vi "C4Buf_writeFeature.vi"(0 "c4buf in":refnum<k24>, 5 "name in":string, 7 "value in":string, 11 "error in":errorcluster) -> (4 "c4buf out":refnum<k24>, 15 "error out":errorcluster)   [LabVIEW 2015, in "libC4HdlLV.lvlib"]
uses:
  libC4HdlLV.lvlib
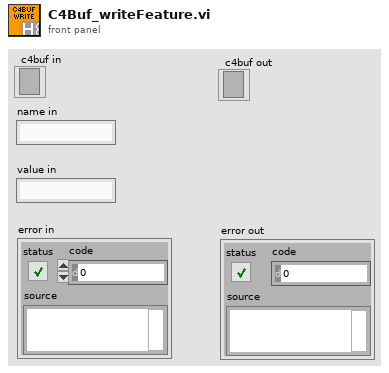
[diagram p1: front panel]
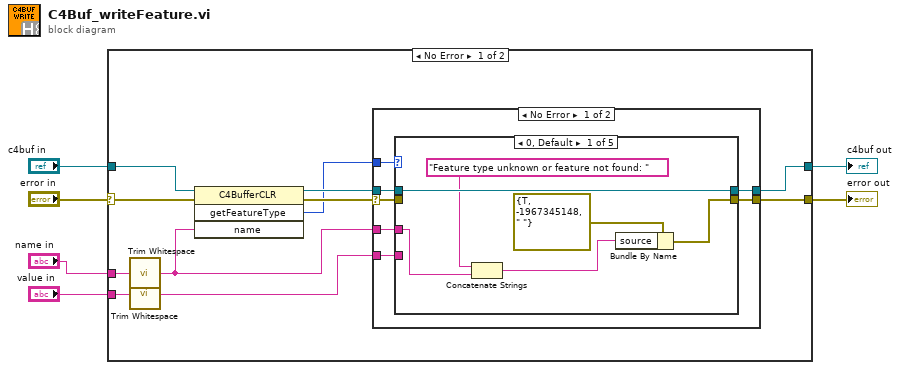
[diagram p0: block diagram]
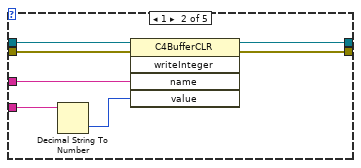
[diagram p2: hidden frame]
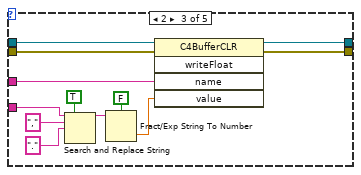
[diagram p3: hidden frame]
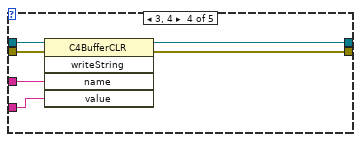
[diagram p4: hidden frame]
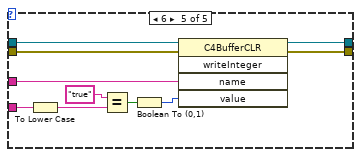
[diagram p5: hidden frame]
diagram:
  n1 = case shown="No Error" "error in" {
    selector: "error in" -> [w11 w69]
    tunnel: [w16 w68] -> w1
    tunnel: [w15 w69] -> w2
    tunnel: "name in" -> [w14 _]
    tunnel: "c4buf in" -> [w12 w68]
    tunnel: "value in" -> [w10 _]
    frame No Error {
      n2 = call <vilib>:"Trim Whitespace.vi"("string"=w14) -> ("trimmed string"=w9:string)  [unwired: 1 in]
      n3 = call <vilib>:"Trim Whitespace.vi"("string"=w10) -> ("trimmed string"=w13:string)  [unwired: 1 in]
      n4 = invoke class="C4BufferCLR" method="getFeatureType"(reference=w12, error in=w11, "name"=w9) -> (reference out=w17:refnum<k24>, error out=w8:errorcluster, "getFeatureType"=w7:i64)  [unwired: 1 in, 1 out]
      n5 = case shown="No Error" w8 {
        selector: w8 -> [w19 w67]
        tunnel: w17 -> [w24 w66]
        tunnel: [w23 w66] -> w16
        tunnel: [w22 w67] -> w15
        tunnel: w13 -> [w21 _]
        tunnel: w9 -> [w20 _]
        tunnel: w7 -> [w18 _]
        frame No Error {
          n6 = case shown="0, Default" w18 {
            tunnel: w24 -> [w30 w37 w49 w55 w65]
            tunnel: w19 -> [_ w36 w48 w54 w64]
            tunnel: w20 -> [w27 w33 w46 w53 w63]
            tunnel: w21 -> [_ w35 w42 w50 w60]
            tunnel: [w30 w32 w45 w52 w62] -> w23
            tunnel: [w25 w31 w44 w51 w61] -> w22
            frame 0, Default {
              n7 = Concatenate Strings("Feature type unknown or feature not found: " ("source"), w27) -> (w29:string)
              n8 = Bundle By Name(cluster=errorcluster {"status"=TRUE, "code"=-1967345148, "source"=" "} ("error out"), "source"=w29) -> (w25:errorcluster)
            }
            frame 1 {
              n9 = Decimal String To Number(string=w35) -> (number=w34:i32)  [unwired: 2 in, 1 out]
              n10 = invoke class="C4BufferCLR" method="writeInteger"(reference=w37, error in=w36, "name"=w33, "value"=w34) -> (reference out=w32:refnum<k24>, error out=w31:errorcluster)  [unwired: 1 in, 3 out]
            }
            frame 2 {
              n11 = Search and Replace String(replace all?=TRUE ("replace all? (F)"), input string=w42, search string=",", replace string="." ("replace string (\"\")")) -> (result string=w41:string)  [unwired: 4 in, 3 out]
              n12 = Fract/Exp String To Number(use system decimal point (T)=FALSE, string=w41) -> (number=w47:dbl)  [unwired: 2 in, 1 out]
              n13 = invoke class="C4BufferCLR" method="writeFloat"(reference=w49, error in=w48, "name"=w46, "value"=w47) -> (reference out=w45:refnum<k24>, error out=w44:errorcluster)  [unwired: 1 in, 3 out]
            }
            frame 3, 4 {
              n14 = invoke class="C4BufferCLR" method="writeString"(reference=w55, error in=w54, "name"=w53, "value"=w50) -> (reference out=w52:refnum<k24>, error out=w51:errorcluster)  [unwired: 1 in, 3 out]
            }
            frame 6 {
              n15 = To Lower Case(string=w60) -> (all lower case string=w59:string)
              n16 = Equal?(x="true", y=w59) -> (x = y?=w56:bool)
              n17 = Boolean To (0,1)(Boolean=w56) -> (0, 1=w57:i16)
              n18 = invoke class="C4BufferCLR" method="writeInteger"(reference=w65, error in=w64, "name"=w63, "value"=w57) -> (reference out=w62:refnum<k24>, error out=w61:errorcluster)  [unwired: 1 in, 3 out]
            }
          }
        }
        frame Error {
        }
      }
    }
    frame Error {
    }
  }
  "error out" <- w2
  "c4buf out" <- w1
